vi "PYTHON Test Script Node.vi"() -> ()   [LabVIEW 2011]
panel:
  out "version":string
  in  "error in (no error)":errorcluster
  out "out (really a float)":string
  in  "div":dbl=9.0 format="%.2f"
  out "num":dbl format="%.6f"
  out "error out":errorcluster
  out "result":string="Python is cool!!!!!!"
  in  "Text":string="Hello brave World!\r"
  in  "val":dbl=4.0 format="%.2f"
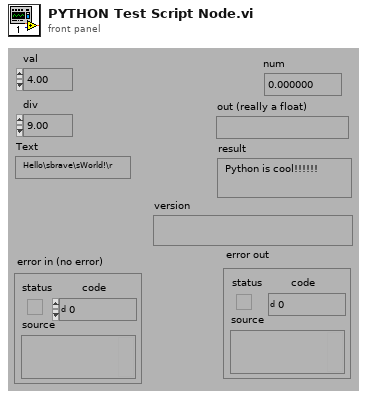
[diagram p1: front panel]
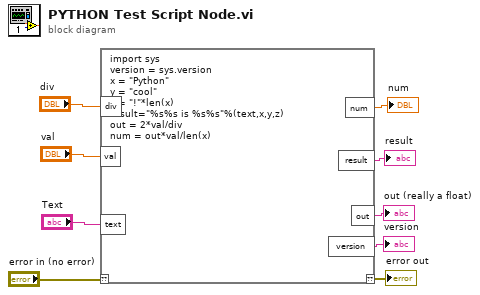
[diagram p0: block diagram]
diagram:
  n1 = script code="import sys\nversion = sys.version\nx = \"Python\"\ny = \"cool\"\nz = \"!\"*len(x)\nresult=\"%s%s is %s%s\"%(text,x,y,z)\nout = 2*val/div\nnum = out*val/len(x)"("??"="error in (no error)", "val"="val", "text"="Text", "div"="div") -> ("??"=→"error out":errorcluster, "out"=→"out (really a float)":string, "result"=→"result":string, "num"=→"num":dbl, "version"=→"version":string)
